vi "PIDControllers (SubVI).vi"(0 "HMI-10HIC200":dbl, 1 "HMI-10LIC200_MA":bool, 2 "BPCS-10LI200":dbl, 3 "HMI-10LIC200-SP":dbl, 5 "HMI-10LIC200-KPID":dbl[](array[numeric]), 7 "HMI-10TIC100-SP":dbl, 9 "BPCS-10TI100":dbl, 11 "HMI-10HIC300":dbl, 12 "HMI-10TIC100_MA":bool, 13 "HMI-10HIC100":dbl, 14 "HMI-10TIC100-KPID":dbl[](array[numeric])) -> (4 "BPCS-10Y200":dbl format="%.2f", 6 "BPCS-SIM-TX-ARRAY":dbl[](array[numeric]), 8 "BPCS-10AY300":dbl, 10 "BPCS-10TY100":dbl format="%.2f")   [LabVIEW 2018]
uses:
  <vilib>/addons/control/pid/pid.llb/PID Advanced (DBL).vi
  <vilib>/addons/control/pid/NI_PID_pid.lvlib
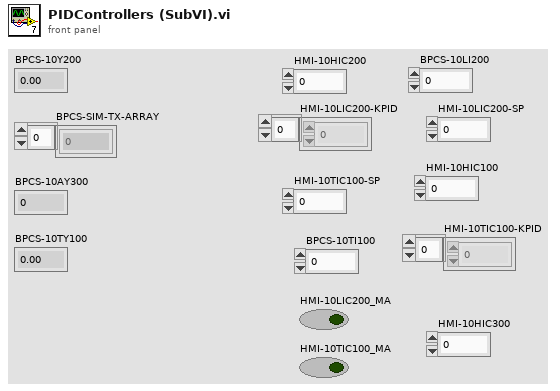
[diagram p1: front panel]
types:
  T1 = cluster{"HMI-10LIC200-KPID[0]":dbl, "HMI-10LIC200-KPID[1]":dbl, "HMI-10LIC200-KPID[2]":dbl}
  T2 = cluster{"HMI-10TIC100-KPID[0]":dbl, "HMI-10TIC100-KPID[1]":dbl, "HMI-10TIC100-KPID[2]":dbl}
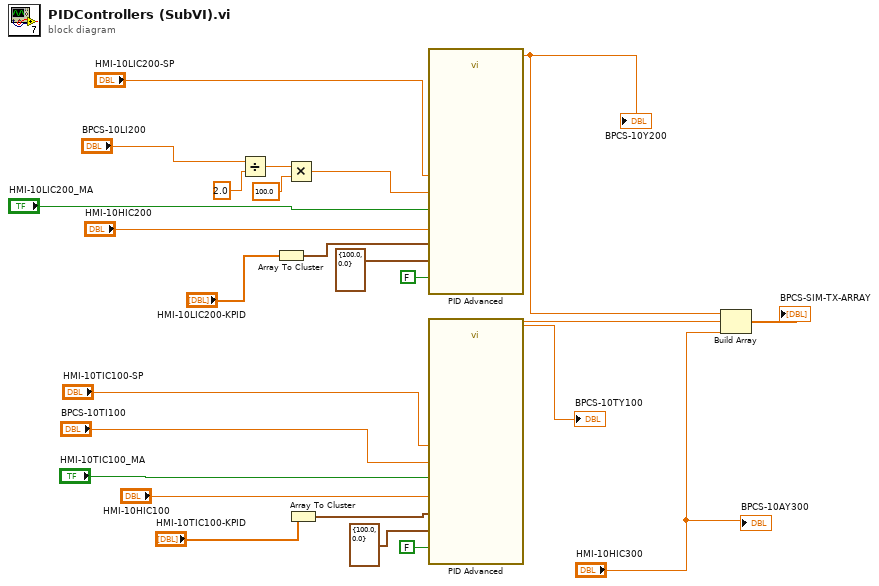
[diagram p0: block diagram]
diagram:
  n1 = Divide(x="BPCS-10LI200", y=2.0 ("x")) -> (x/y=w3:dbl)
  n2 = Array To Cluster(array="HMI-10LIC200-KPID") -> (cluster=w6:T1)
  n3 = Multiply(x=w3, y=100.0) -> (x*y=w5:dbl)
  n4 = Array To Cluster(array="HMI-10TIC100-KPID") -> (cluster=w9:T2)
  n5 = call-poly <vilib>:"PID Advanced.vi"("setpoint"="HMI-10LIC200-SP", "output range"=cluster{"output high":dbl, "output low":dbl} {"output high"=100.0, "output low"=0.0}, "auto? (T)"="HMI-10LIC200_MA", "manual control"="HMI-10HIC200", "process variable"=w5, "PID gains"=w6, "reinitialize? (F)"=FALSE) -> ("output"=w14:dbl)  [unwired: 7 in, 1 out]
  "BPCS-10Y200" <- w14
  n6 = call-poly <vilib>:"PID Advanced.vi"("setpoint"="HMI-10TIC100-SP", "output range"=cluster{"output high":dbl, "output low":dbl} {"output high"=100.0, "output low"=0.0}, "auto? (T)"="HMI-10TIC100_MA", "manual control"="HMI-10HIC100", "process variable"="BPCS-10TI100", "PID gains"=w9, "reinitialize? (F)"=FALSE) -> ("output"=w15:dbl)  [unwired: 7 in, 1 out]
  "BPCS-10TY100" <- w15
  n7 = Build Array(w14, w15, "HMI-10HIC300") -> (→"BPCS-SIM-TX-ARRAY":dbl[])
  "BPCS-10AY300" <- "HMI-10HIC300"
